vi "Write DataLogObjectvi.vi"(8 "error in (no error)":errorcluster, 10 "DataLogging.lvclass":refnum<class "DataLogging.lvclass">, 11 "Analysis in":refnum<class "Analysis.lvclass">) -> (0 "error out":errorcluster, 3 "Analysis out":refnum<class "Analysis.lvclass">)   [LabVIEW 2017, in "Analysis.lvclass"]
uses:
  Analysis.lvclass
  DataLoggingText/DataLogging.lvclass
  Analysis.lvclass/Analysis.ctl
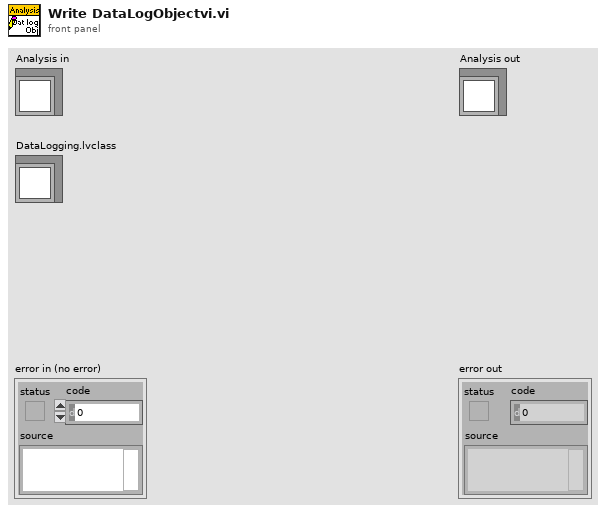
[diagram p1: front panel]
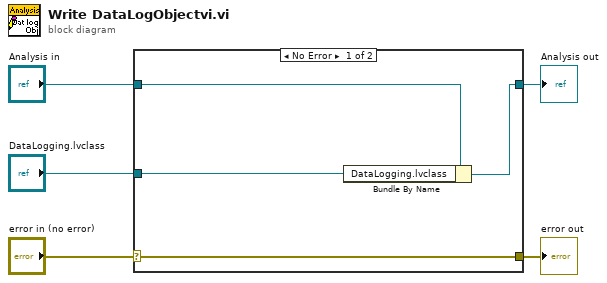
[diagram p0: block diagram]
diagram:
  n1 = case shown="No Error" "error in (no error)" {
    selector: "error in (no error)" -> [w9 w10]
    tunnel: [w9 w10] -> w4
    tunnel: [w7 w11] -> w2
    tunnel: "Analysis in" -> [w8 w11]
    tunnel: "DataLogging.lvclass" -> [w6 _]
    frame No Error {
      n2 = Bundle By Name(cluster=w8, "DataLogging.lvclass"=w6) -> (w7:refnum<class "Analysis.lvclass">)
    }
    frame Error {
    }
  }
  "error out" <- w4
  "Analysis out" <- w2
